vi "tm_getframe_a.vi"(8 "error in (no error)":errorcluster {"code" format="%.0x"}, 9 "Frame Index":i32=-1, 10 "Buffer Info":T1, 11 "Handle in":u32) -> (0 "error out":errorcluster {"code" format="%.0x"}, 1 "Data 8":u8[][](array[numeric]), 2 "Data 16":u16[][](array[numeric]), 3 "Handle out":u32, 4 "Electron Info":cluster{"coefficient":sgl, "offset":sgl})   [LabVIEW 2021]
uses:
  tmcamcon.dll
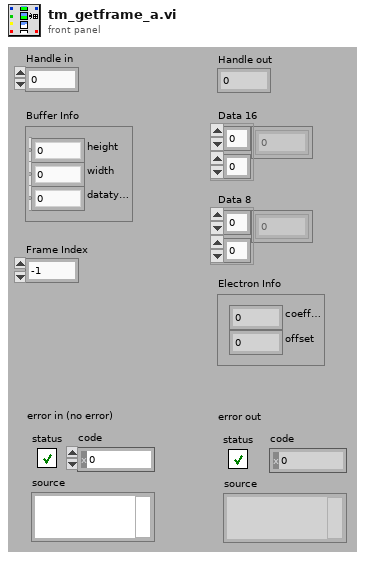
[diagram p1: front panel]
types:
  T1 = cluster{"height":u32, "width":u32, "datatype":u32}
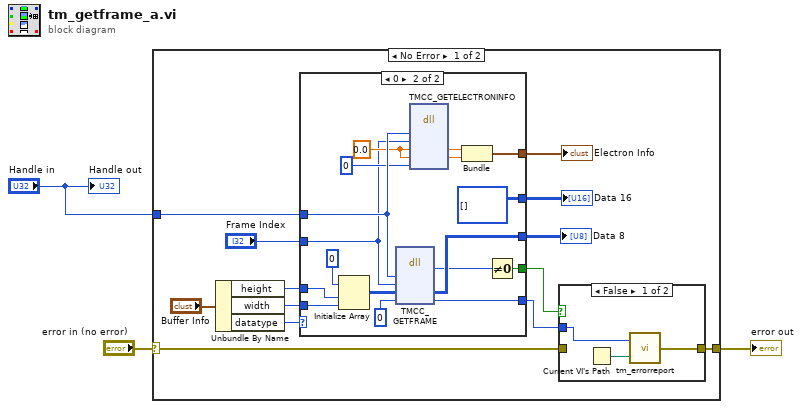
[diagram p0: block diagram]
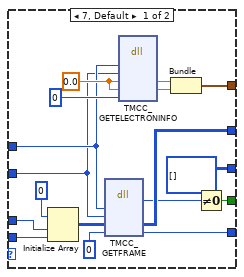
[diagram p3: hidden frame]
diagram:
  n1 = case shown="No Error" "error in (no error)" {
    selector: "error in (no error)" -> [w7 w55]
    tunnel: [w6 w55] -> w2
    tunnel: "Handle in" -> [w16 _]
    frame No Error {
      n2 = Unbundle By Name("Buffer Info") -> ("height"=w11:u32, "width"=w10:u32, "datatype"=w9:u32)
      n3 = case shown="0" w9 {
        tunnel: w11 -> [w36 w53]
        tunnel: w10 -> [w35 w52]
        tunnel: w16 -> [w24 w46]
        tunnel: "Frame Index" -> [w23 w40]
        tunnel: [w32 w49] -> w5
        tunnel: [w21 w39] -> w4
        tunnel: [u8[][] [] ("Data 8") w47] -> w14
        tunnel: [w30 u16[][] [] ("Data 16")] -> w13
        tunnel: [w29 w41] -> w8
        frame 7, Default {
          w26 = sgl 0.0 ("C")
          n4 = Initialize Array(u16 0, w36, w35) -> (w33:u16[][])
          n5 = dll-call lib="tmcamcon.dll" fn="TMCC_GETFRAME"("index"=w24, "frameindex"=w23, "imgarray"=w33, "Erval"=0) -> ("return type"=w22:u32, "imgarray"=w30:u16[][], "Erval"=w32:i32)  [unwired: 5 in, 2 out]
          n6 = dll-call lib="tmcamcon.dll" fn="TMCC_GETELECTRONINFO"("index"=w24, "frame"=w23, "C"=w26, "O"=w26, "Erval"=0) -> ("C"=w28:sgl, "O"=w27:sgl)  [unwired: 7 in, 2 out]
          n7 = Bundle("C"=w28, "O"=w27) -> (w29:cluster{"C":sgl, "O":sgl})  [unwired: 1 in]
          n8 = Not Equal To 0?(x=w22) -> (x != 0?=w21:bool)
        }
        frame 0 {
          w42 = sgl 0.0 ("C")
          n9 = Initialize Array(u8 0, w53, w52) -> (w50:u8[][])
          n10 = dll-call lib="tmcamcon.dll" fn="TMCC_GETFRAME"("index"=w46, "frameindex"=w40, "imgarray"=w50, "Erval"=0) -> ("return type"=w38:u32, "imgarray"=w47:u8[][], "Erval"=w49:i32)  [unwired: 5 in, 2 out]
          n11 = dll-call lib="tmcamcon.dll" fn="TMCC_GETELECTRONINFO"("index"=w46, "frame"=w40, "C"=w42, "O"=w42, "Erval"=0) -> ("C"=w45:sgl, "O"=w44:sgl)  [unwired: 7 in, 2 out]
          n12 = Bundle("C"=w45, "O"=w44) -> (w41:cluster{"C":sgl, "O":sgl})  [unwired: 1 in]
          n13 = Not Equal To 0?(x=w38) -> (x != 0?=w39:bool)
        }
      }
      "Data 16" <- w13
      "Data 8" <- w14
      "Electron Info" <- w8
      n14 = case shown="False" w4 {
        tunnel: w7 -> [_ w20]
        tunnel: [w18 w20] -> w6
        tunnel: w5 -> [w17 _]
        frame False {
          n15 = Current VI's Path() -> (path=w19:path)
          n16 = call <userlib>:"tm_errorreport.vi"("Source"=w19, "Error"=w17) -> ("error out"=w18:errorcluster)
        }
        frame True {
        }
      }
    }
    frame Error {
    }
  }
  "error out" <- w2
  "Handle out" <- "Handle in"
